vi "GCliTemplate.vi"(6 "GUI Mode? {F)":bool, 8 "error in (no error)":errorcluster) -> (0 "error out":errorcluster)   [LabVIEW 2019, in "Hawkeye.lvlib"]
uses:
  Hawkeye.lvlib
  <vilib>/Wiresmith Technology/G CLI/CLI Class/CLI.lvclass
panel:
  in  "Tab Control":enum32{"GUI Mode", "CLI Mode"}(tab)
  in  "Output File Path":path=path "E:/sw-deps-monitor/changed-files.txt"
  in  "Input 2":string="initial-ci-check-yml"
  in  "Input 1":string="main"
  in  "PathInput":path=path "E:/sw-deps-monitor"
  out "Args":string[](array[string])=["Arg1", "Arg2"]
  # "When in GUI Mode, the controls will be used, \nin CLI Mode the Args will be used"
  # "Workspace path Input"
  # "Input 1"
  # "Input 2"
  # "Output File Path"
  # "Command to run the VI from terminal\ng-cli -v --lv-ver 2023 --arch 32 \"E:\\sw-deps-monitor\\CICD\\Reusables\\GCliTemplate.vi\" -- \"Arg1\" \"Arg2\""
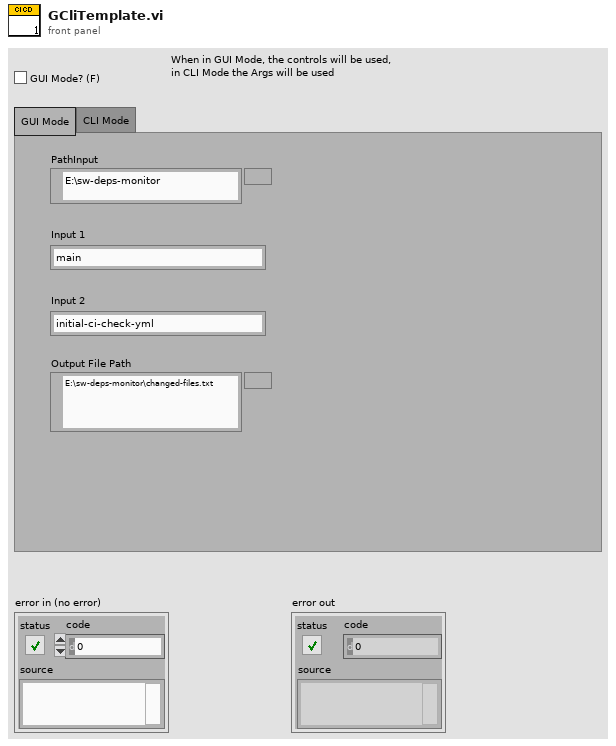
[diagram p1: front panel]
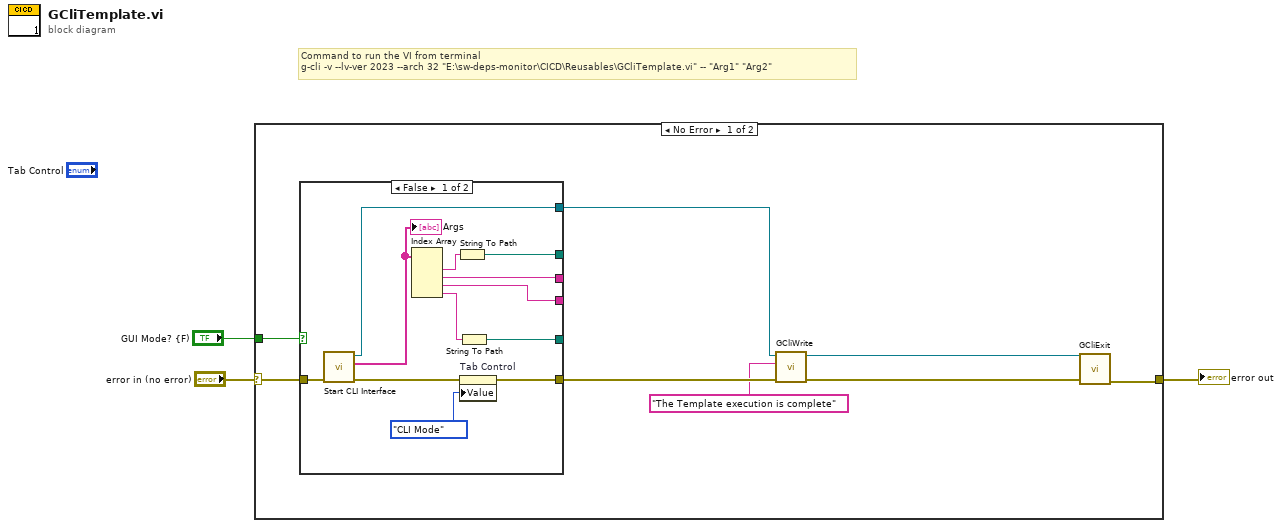
[diagram p0: block diagram]
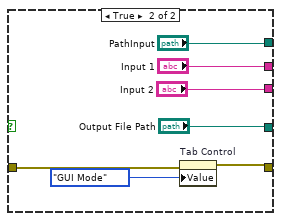
[diagram p2: hidden frame]
diagram:
  # "Command to run the VI from terminal\ng-cli -v --lv-ver 2023 --arch 32 \"E:\\sw-deps-monitor\\CICD\\Reusables\\GCliTemplate.vi\" -- \"Arg1\" \"Arg2\""
  n1 = case shown="No Error" "error in (no error)" {
    selector: "error in (no error)" -> [w10 w31]
    tunnel: "GUI Mode? {F)" -> [w11 _]
    tunnel: [w5 w31] -> w1
    frame No Error {
      n2 = case shown="False" w11 {
        tunnel: [w22 "Input 1"] -> _
        tunnel: [w19 "PathInput"] -> _
        tunnel: [w18 "Output File Path"] -> _
        tunnel: [w21 "Input 2"] -> _
        tunnel: w10 -> [w15 w26]
        tunnel: [w17 w25] -> w9
        tunnel: [w13 _] -> w6
        frame False {
          n3 = call <vilib>:"Start CLI Interface.vi"("error in (no error)"=w15) -> ("error out"=w14:errorcluster, "Custom Parameters"=w12:string[], "CLI out"=w13:refnum<class "CLI.lvclass">)  [unwired: 7 in, 1 out]
          "Args" <- w12
          n4 = Index Array(array=w12) -> (element #1=w23:string, element #2=w22:string, element #3=w21:string, element #4=w20:string)  [unwired: 4 in]
          n5 = String To Path(string=w23) -> (path=w19:path)
          n6 = String To Path(string=w20) -> (path=w18:path)
          n7 = property on="Tab Control" class="TabCtl (strict)"(error in=w14, "Value"=enum32{"GUI Mode", "CLI Mode"}."CLI Mode" ("Tab Control")) -> (error out=w17:errorcluster)  [unwired: 1 in, 1 out]
        }
        frame True {
          n8 = property on="Tab Control" class="TabCtl (strict)"(error in=w26, "Value"=enum32{"GUI Mode", "CLI Mode"}."GUI Mode" ("Tab Control")) -> (error out=w25:errorcluster)  [unwired: 1 in, 1 out]
        }
      }
      n9 = call "GCliWrite.vi"("error in (no error)"=w9, "Text to Write"="The Template execution is complete", "CLI in"=w6) -> ("error out"=w8:errorcluster, "CLI out"=w7:refnum<class "CLI.lvclass">)  [unwired: 7 in]
      n10 = call "GCliExit.vi"("error in (no error)"=w8, "CLI in"=w7) -> ("error out"=w5:errorcluster)  [unwired: 9 in]
    }
    frame Error {
    }
  }
  "error out" <- w1
